vi "Initial Values-format and values-Ref plots window.vi"() -> (13 "Values.Boolean":bool[](array[boolean]), 14 "Keys setup.DBL":T2=[{"key"="Control FPGA.Clock Freq (MHz)", "Save?"=TRUE, "Default"=240.0}, {"key"="DAQ FPGA.Clock Freq (MHz)", "Save?"=TRUE, "Default"=240.0}], 15 "Values.DBL":dbl[](array[numeric]), 16 "Keys setup.String":T3=[{"key"="Control FPGA.MAC address", "Save?"=TRUE, "Default"="AABBCCDDEEFF"}, {"key"="DAQ FPGA.Target", "Save?"=TRUE, "Default"="RIO0"}, {"key"="XY Stage.COM port", "Save?"=TRUE, "Default"="COM7"}, {"key"="DAQmx Chan.Pockels Control", "Save?"=TRUE, "Default"=""}, {"key"="DAQmx Chan.Hard Shutter", "Save?"=TRUE, "Default"=""}, {"key"="DAQmx Chan.PMT 1", "Save?"=TRUE, "Default"=""}, {"key"="DAQmx Chan.PMT 2", "Save?"=TRUE, "Default"=""}, {"key"="DAQmx Chan.Encoder Trigger", "Save?"=TRUE, "Default"=""}, {"key"="DAQmx Chan.Optional Trigger 1", "Save?"=TRUE, "Default"=""}, {"key"="DAQmx Chan.Optional Trigger 2", "Save?"=TRUE, "Default"=""}, {"key"="DAQmx Chan.Optional Trigger 3", "Save?"=TRUE, "Default"=""}], 17 "Values.Strings":string[](array[string]), 18 "Keys setup.Boolean":T1, 19 "error out":errorcluster)   [LabVIEW 2017]
uses:
  Typedefs/Ini file interface (String).ctl
  Typedefs/Ini file interface (DBL).ctl
  Typedefs/Ini file interface (Boolean).ctl
  User Interface/Globals/gl_Windows Ctrl refs.vi
panel:
  # "NOTES:\n1. \"Control FPGA.Ethernet port\" is detected automatically. It is not saved/loaded from file.\n2. \"Control FPGA.Ethernet Opened\" is detected automatically. It is not saved/loaded from file."
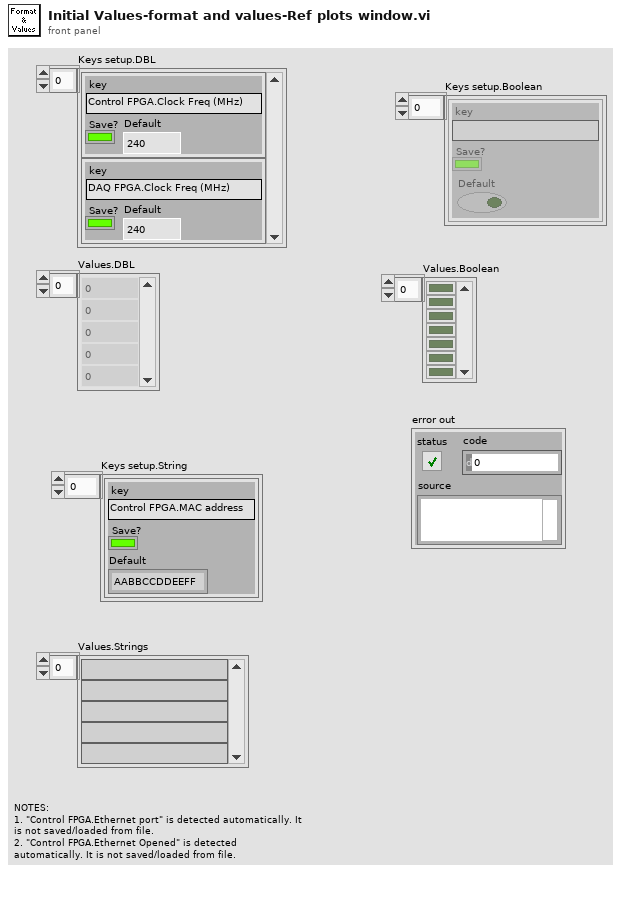
[diagram p1: front panel]
types:
  T1 = typedef "Ini file interface (Boolean).ctl" = cluster{"key":string, "Save?":bool, "Default":bool}[]
  T2 = typedef "Ini file interface (DBL).ctl" = cluster{"key":string, "Save?":bool, "Default":dbl}[]
  T3 = typedef "Ini file interface (String).ctl" = cluster{"key":string, "Save?":bool, "Default":string}[]
  T4 = typedef "Reference plots window ctrl refs.ctl" = cluster{"Refresh rate (ms)":refnum<vi>, "Buffer Size":refnum<vi>}
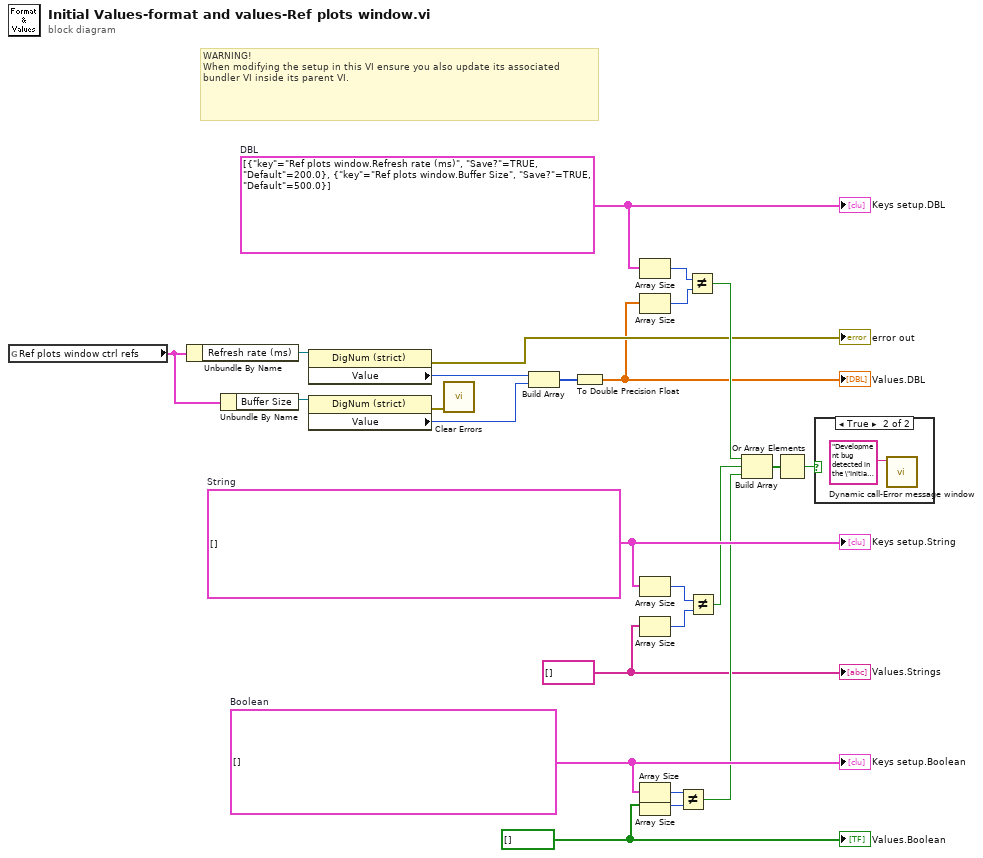
[diagram p0: block diagram]
diagram:
  w4 = T2 [{"key"="Ref plots window.Refresh rate (ms)", "Save?"=TRUE, "Default"=200.0}, {"key"="Ref plots window.Buffer Size", "Save?"=TRUE, "Default"=500.0}]  # DBL
  w12 = string[] [] ("appended array")
  w13 = bool[] [] ("appended array")
  w24 = T1 []  # Boolean
  w25 = T3 []  # String
  # "WARNING!\nWhen modifying the setup in this VI ensure you also update its associated bundler VI inside its parent VI."
  n1 = global read "gl_Windows Ctrl refs.vi" "Ref plots window ctrl refs"() -> (w7:T4)
  n2 = Unbundle By Name(w7) -> ("Refresh rate (ms)"=w6:refnum<vi>)
  n3 = Unbundle By Name(w7) -> ("Buffer Size"=w5:refnum<vi>)
  n4 = property class="DigNum (strict)"(reference=w6) -> (error out=→"error out":errorcluster, "Value"=w10:u32)  [unwired: 1 in, 1 out]
  n5 = property class="DigNum (strict)"(reference=w5) -> (error out=w8:errorcluster, "Value"=w9:i32)  [unwired: 1 in, 1 out]
  n6 = call <vilib>:"Clear Errors.vi"("error in (no error)"=w8) -> ()  [unwired: 5 in, 2 out]
  n7 = Build Array(w10, w9) -> (w11:u32[])
  n8 = To Double Precision Float(number=w11) -> (double precision float=w2:dbl[])
  "Values.DBL" <- w2
  n9 = Array Size(array=w4) -> (size(s)=w21:i32)
  n10 = Array Size(array=w2) -> (size(s)=w20:i32)
  n11 = Array Size(array=w25) -> (size(s)=w23:i32)
  n12 = Array Size(array=w12) -> (size(s)=w22:i32)
  n13 = Array Size(array=w24) -> (size(s)=w19:i32)
  n14 = Array Size(array=w13) -> (size(s)=w18:i32)
  n15 = Not Equal?(x=w19, y=w18) -> (x != y?=w16:bool)
  n16 = Not Equal?(x=w21, y=w20) -> (x != y?=w15:bool)
  n17 = Not Equal?(x=w23, y=w22) -> (x != y?=w14:bool)
  n18 = Build Array(w15, w14, w16) -> (w17:bool[])
  n19 = Or Array Elements(Boolean array=w17) -> (logical OR=w1:bool)
  n20 = case shown="True" w1 {
    frame False {
    }
    frame True {
      n21 = call "Dynamic call-Error message window.vi"("Error Message"="Development bug detected in the \"Initial Values-format and values-Ref window.vi\".\nPlease correct the set up in this VI.") -> ()  [unwired: 10 in, 1 out]
    }
  }
  "Keys setup.String" <- w25
  "Keys setup.DBL" <- w4
  "Values.Strings" <- w12
  "Keys setup.Boolean" <- w24
  "Values.Boolean" <- w13
